vi "Update Debug Panel.vi"(8 "error in (no error)":errorcluster, 10 "Module Action":string, 11 "Rename in":refnum<class "Rename.lvclass">) -> (0 "error out":errorcluster, 3 "Rename out":refnum<class "Rename.lvclass">)   [LabVIEW 2015, in "Generic Module Library.lvlib" / "Template G_Module.lvlib" / "Rename.lvclass"]
uses:
  Rename.lvclass
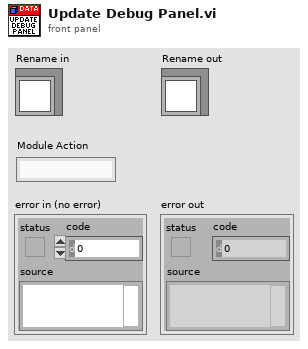
[diagram p1: front panel]
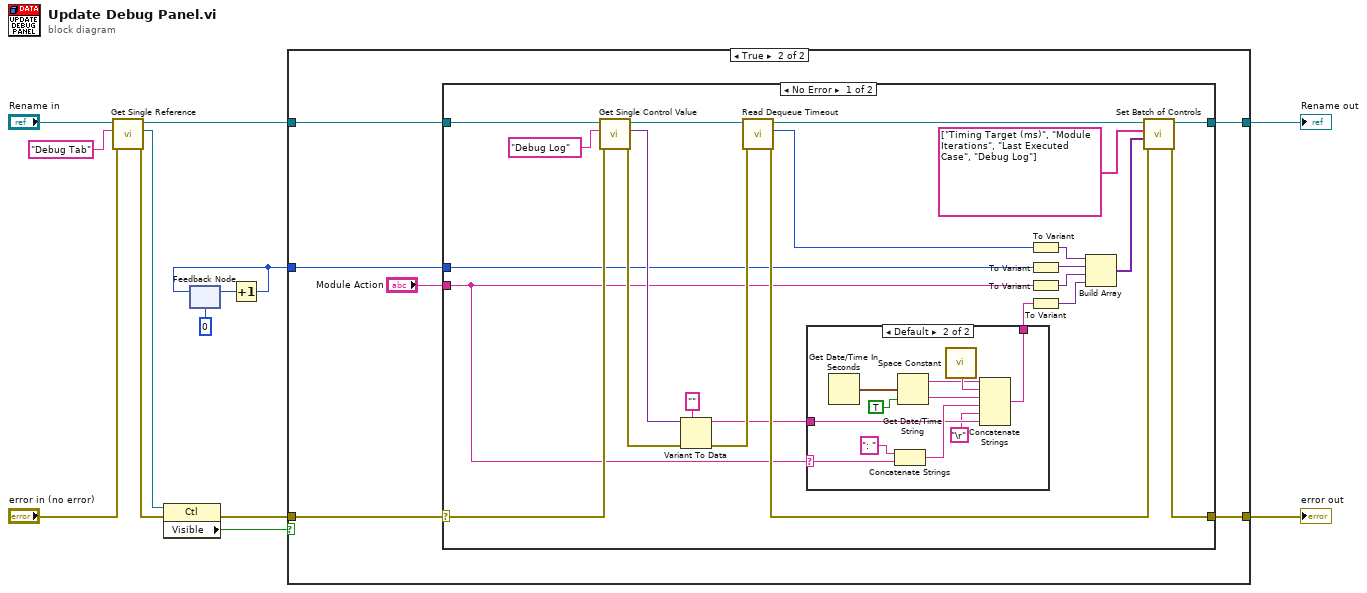
[diagram p0: block diagram]
diagram:
  n1 = call "Get Single Reference.vi"("error in (no error)"="error in (no error)", "Control Name"="Debug Tab", "Rename in"="Rename in") -> ("error out"=w7:errorcluster, "Control Reference"=w8:refnum<vi>, "Rename out"=w10:refnum<class "Rename.lvclass">)  [unwired: 6 in]
  n2 = property class="Ctl"(reference=w8, error in=w7) -> (error out=w6:errorcluster, "Visible"=w5:bool)  [unwired: 1 out]
  n3 = feedback #1(u64 0) -> (w2:u64)
  n4 = Increment(x=w2) -> (x+1=w1:u64)
  n5 = feedback-in #1(w1) -> ()
  n6 = case shown="True" w5 {
    tunnel: [w14 w21] -> w13
    tunnel: [w15 w20] -> w12
    tunnel: w10 -> [w15 w18]
    tunnel: w6 -> [w14 w17]
    tunnel: w1 -> [_ w16]
    frame False {
    }
    frame True {
      n7 = case shown="No Error" w17 {
        selector: w17 -> [w30 w58]
        tunnel: [w39 w58] -> w21
        tunnel: [w40 w57] -> w20
        tunnel: w18 -> [w32 w57]
        tunnel: "Module Action" -> [w23 _]
        tunnel: w16 -> [w22 _]
        frame No Error {
          n8 = call "Get Single Control Value.vi"("error in (no error)"=w30, "Control Name"="Debug Log", "Rename in"=w32) -> ("error out"=w29:errorcluster, "Value"=w26:variant, "Rename out"=w31:refnum<class "Rename.lvclass">)  [unwired: 6 in]
          n9 = Variant To Data(error in=w29, type="", Variant=w26) -> (data=w25:string, error out=w27:errorcluster)
          n10 = call-dynamic "Read Dequeue Timeout.vi"("error in (no error)"=w27, "Rename in"=w31) -> ("error out"=w37:errorcluster, "Dequeue Timeout"=w36:i32, "Rename out"=w38:refnum<class "Rename.lvclass">)  [unwired: 7 in]
          n11 = case shown="Default" w23 {
            selector: w23 -> [_ w51]
            tunnel: [w45 w55] -> w34
            tunnel: w25 -> [w45 w48]
            frame "Timeout" {
            }
            frame Default {
              n12 = Get Date/Time In Seconds() -> (seconds since 1Jan1904=w56:timestamp)
              n13 = Concatenate Strings(": " ("string"), w51) -> (w49:string)
              n14 = Get Date/Time String(seconds (now)=w56, want seconds? (F)=TRUE) -> (date string=w52:string, time string=w54:string)  [unwired: 1 in]
              n15 = call <vilib>:"Space Constant.vi"() -> ("String"=w53:string)
              n16 = Concatenate Strings(w52, w53, w54, w49, "\r", w48) -> (w55:string)
            }
          }
          n17 = To Variant(anything=w36) -> (Variant=w35:variant)
          n18 = To Variant(anything=w22) -> (Variant=w42:variant)
          n19 = To Variant(anything=w23) -> (Variant=w43:variant)
          n20 = To Variant(anything=w34) -> (Variant=w33:variant)
          n21 = Build Array(w35, w42, w43, w33) -> (w41:variant[])
          n22 = call "Set Batch of Controls.vi"("error in (no error)"=w37, "Indicator Values"=w41, "Indicator Names"=string[] ["Timing Target (ms)", "Module Iterations", "Last Executed Case", "Debug Log"], "Rename in"=w38) -> ("error out"=w39:errorcluster, "Rename out"=w40:refnum<class "Rename.lvclass">)  [unwired: 6 in]
        }
        frame Error {
        }
      }
    }
  }
  "error out" <- w13
  "Rename out" <- w12
